vi "IOL Sensor Value Invalid 6001--error.vi"(11 "Sensor Key":string) -> (0 "error out":errorcluster)   [LabVIEW 2024, in "IOLink.lvlib"]
uses:
  IOLink.lvlib
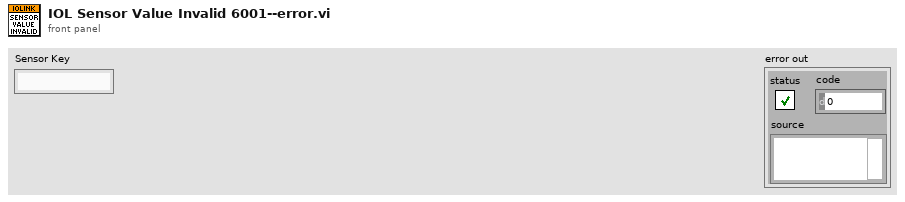
[diagram p1: front panel]
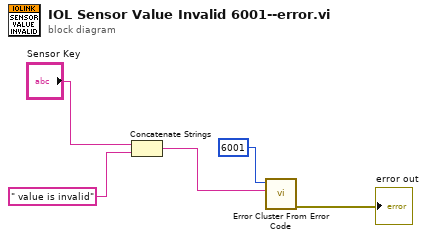
[diagram p0: block diagram]
diagram:
  n1 = Concatenate Strings("Sensor Key", " value is invalid" ("string")) -> (w3:string)
  n2 = call <vilib>:"Error Cluster From Error Code.vi"("error message (\"\")"=w3, "error code (0)"=6001) -> ("error out"=→"error out":errorcluster)  [unwired: 7 in]
